vi "update mc lsitbox from stim config (subVI).vi"(6 "off string (\"-\")":string="-", 7 "description []":string[](array[string]), 8 "error in (no error)":errorcluster, 9 "string stim. matrix":string[][](array[string]), 10 "bool stim. matrix":bool[][](array[boolean]), 11 "mc listbox refnum":refnum<vi>) -> (0 "error out":errorcluster, 3 "mc listbox refnum out":refnum<vi>)   [LabVIEW 2021]
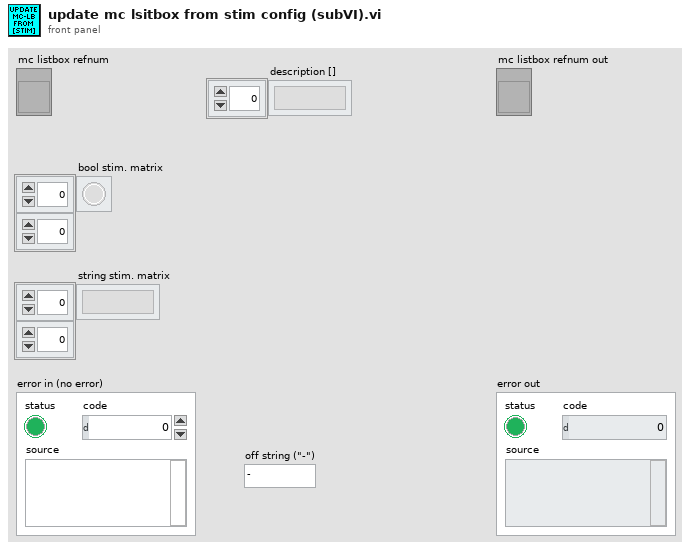
[diagram p1: front panel]
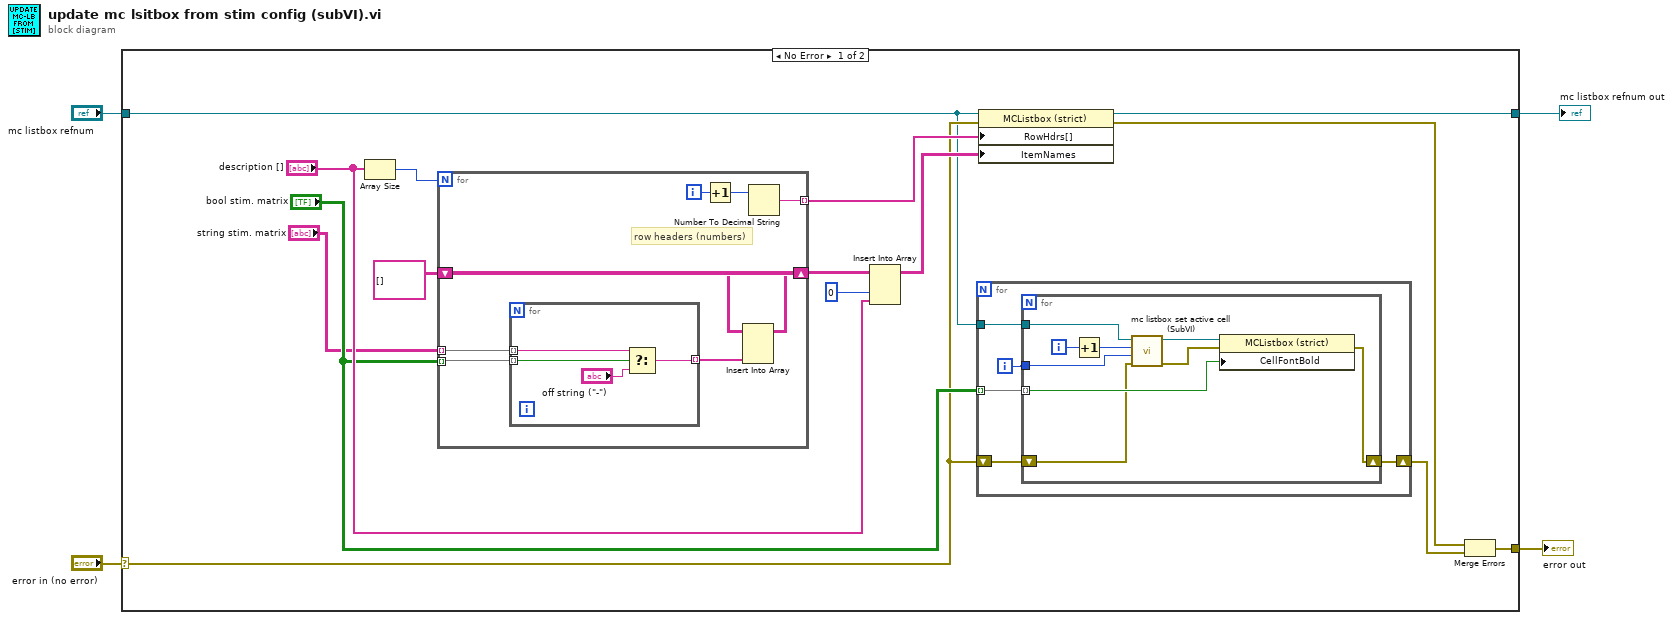
[diagram p0: block diagram]
diagram:
  n1 = case shown="No Error" "error in (no error)" {
    selector: "error in (no error)" -> [w9 w46]
    tunnel: "mc listbox refnum" -> [w8 w47]
    tunnel: [w7 w46] -> w2
    tunnel: [w5 w47] -> w1
    frame No Error {
      n2 = Array Size(array="description []") -> (size(s)=w13:i32)
      n3 = for {
        N: w13 -> [_]
        shift-right: [w40] -> w16
        shift-left: string[][] [] -> [w39]
        tunnel: [w37] -> w14 mode=indexing
        tunnel: "bool stim. matrix" -> [w35] mode=indexing
        tunnel: "string stim. matrix" -> [w34] mode=indexing
        i -> [w38]
        # "row headers (numbers)"
        n4 = for {
          tunnel: [w44] -> w41 mode=indexing
          tunnel: w35 -> [w43] mode=indexing
          tunnel: w34 -> [w42] mode=indexing
          n5 = Select(t=w42, s=w43, f="off string (\"-\")") -> (s? t:f=w44:string)
        }
        n6 = Increment(x=w38) -> (x+1=w36:i32)
        n7 = Insert Into Array(array=w39, new element=w41) -> (w40:string[][])  [unwired: 2 in]
        n8 = Number To Decimal String(number=w36) -> (decimal integer string=w37:string)  [unwired: 1 in]
      }
      n9 = Insert Into Array(array=w16, index (col)=0 ("disabled index (col)"), new element="description []") -> (w12:string[][])  [unwired: 1 in]
      n10 = for {
        shift-right: [w23] -> w18
        shift-left: w9 -> [w22]
        tunnel: "bool stim. matrix" -> [w21] mode=indexing
        tunnel: w8 -> [w20]
        i -> [w24]
        n11 = for {
          tunnel: w24 -> [w29]
          shift-right: [w32] -> w23
          shift-left: w22 -> [w27]
          tunnel: w21 -> [w31] mode=indexing
          tunnel: w20 -> [w26]
          i -> [w33]
          n12 = Increment(x=w33) -> (x+1=w30:i32)
          n13 = call "mc listbox set active cell (SubVI).vi"("error in (no error)"=w27, "row (0)"=w29, "column (0)"=w30, "multicolumn listbox refnum"=w26) -> ("error out"=w25:errorcluster, "multicolumn listbox refnum out"=w28:refnum<vi>)  [unwired: 6 in]
          n14 = property on="Property Node" class="MCListbox (strict)"(reference=w28, error in=w25, "CellFontBold"=w31) -> (error out=w32:errorcluster)  [unwired: 1 out]
        }
      }
      n15 = property on="Property Node" class="MCListbox (strict)"(reference=w8, error in=w9, "RowHdrs[]"=w14, "ItemNames"=w12) -> (reference out=w5:refnum<vi>, error out=w17:errorcluster)
      n16 = Merge Errors(w17, w18) -> (w7:errorcluster)
    }
    frame Error {
    }
  }
  "error out" <- w2
  "mc listbox refnum out" <- w1
